vi "Set Position Params.vi"(8 "error in (no error)":errorcluster, 10 "Position Params":T1 {"max( |Motor Pos - LRF Distance| )" min=0.0}, 11 "VacuumLine Configuration in":refnum<class "VacuumLine Configuration.lvclass">) -> (0 "error out":errorcluster, 3 "VacuumLine Configuration out":refnum<class "VacuumLine Configuration.lvclass">)   [LabVIEW 2016, in "Hardware.lvlib" / "VacuumLine.lvlib" / "VacuumLine Configuration.lvclass"]
uses:
  <userlib>/Common Components/Hardware/Abstract System/VacuumLine/VacuumLine Config/VacuumLine Configuration.lvclass
  <userlib>/Common Components/Hardware/Abstract System/VacuumLine/VacuumLine/VacuumLine Params.ctl
  <userlib>/Common Components/Hardware/Abstract System/VacuumLine/VacuumLine/Valve Complex.ctl
  <userlib>/Common Components/Hardware/Abstract System/VacuumLine/VacuumLine/Logic Cluster.ctl
  <userlib>/Common Components/Hardware/Abstract System/VacuumLine/VacuumLine Config/VacuumLine Configuration.lvclass/VacuumLine Configuration.ctl
  <userlib>/Common Components/Hardware/Abstract System/VacuumLine/VacuumLine/VacuumLine.lvclass/VacuumLine.ctl
  <userlib>/Common Components/Hardware/Abstract System/VacuumLine/VacuumLine/VacuumLine.lvclass
panel:
  # "Pin#"
  # "Location"
  # "Tolerance"
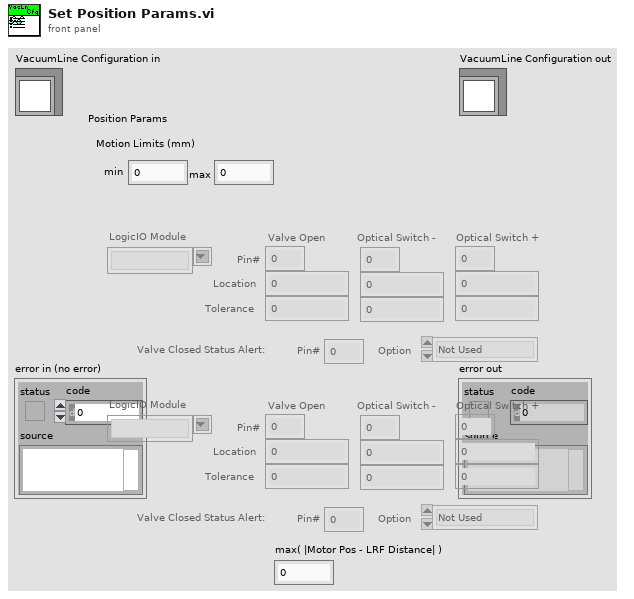
[diagram p1: front panel]
types:
  T1 = typedef "Hardware.lvlib/VacuumLine.lvlib/VacuumLine.lvclass/VacuumLine Params.ctl" = cluster{"Motion Limits":cluster{"min":dbl, "max":dbl}, "Valve Complexes":T2[], "max( |Motor Pos - LRF Distance| )":dbl}
  T2 = typedef "Hardware.lvlib/VacuumLine.lvlib/VacuumLine.lvclass/Valve Complex.ctl" = cluster{"LogicIO Module":string, "Valve Open":T3, "Optical Switch -":T3, "Optical Switch +":T3, "Valve Closed Status Alert":cluster{"Pin#":u8, "Option":enum16{"Not Used", "Normally Closed"}}}
  T3 = typedef "Hardware.lvlib/VacuumLine.lvlib/VacuumLine.lvclass/Logic Cluster.ctl" = cluster{"Pin#":u8, "Location":dbl, "Tolerance":dbl}
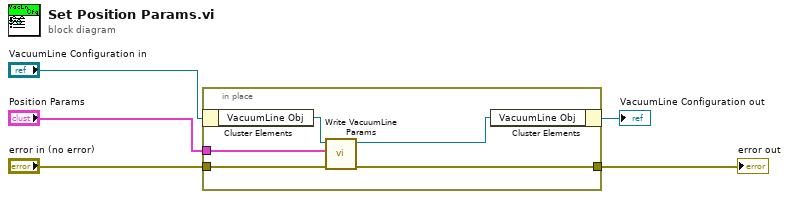
[diagram p0: block diagram]
diagram:
  n1 = in-place {
    in-place-border: "Position Params" -> [w10]
    in-place-border: "error in (no error)" -> [w9]
    in-place-border: [w8] -> w3
    n2 = in-place-cluster #1("VacuumLine Configuration in") -> ("VacuumLine Obj"=w7:refnum<class "VacuumLine.lvclass">)
    n3 = call <userlib>:"Write VacuumLine Params.vi"("error in (no error)"=w9, "Position Params"=w10, "VacuumLine in"=w7) -> ("error out"=w8:errorcluster, "VacuumLine out"=w6:refnum<class "VacuumLine.lvclass">)  [unwired: 7 in]
    n4 = in-place-cluster #1("VacuumLine Obj"=w6) -> (→"VacuumLine Configuration out":refnum<class "VacuumLine Configuration.lvclass">)
  }
  "error out" <- w3
